vi "Lab Panel V5.29.vi"() -> ()   [LabVIEW 2013] (continued)
                  }
                }
              }
              event "RUN LAB01-2": Value Change {
                n578 = event-data() -> ("NewVal"=w843:bool)  [unwired: 1 in, 5 out]
                n579 = local write "run lab01-2"(w843) -> ()
                n580 = case shown="True" w843 {
                  tunnel: w849 -> [_ w887]
                  tunnel: w848 -> [_ w886]
                  tunnel: w846 -> [w851 w885]
                  tunnel: w847 -> [_ w884]
                  tunnel: w845 -> [_ w883]
                  tunnel: [w850 w882] -> w844
                  tunnel: w842 -> [_ w881]
                  tunnel: w841 -> [_ w880]
                  tunnel: w840 -> [_ w879]
                  tunnel: w839 -> [_ w877]
                  frame False {
                    # "stop test"
                    n581 = stacked-sequence {
                      tunnel: w851 -> [w860 _]
                      tunnel: [w852 _] -> w850
                      frame #0 {
                        n582 = local read "DISP LAB01-2"() -> (w859:T4)
                        n583 = Unbundle(w859) -> ("CYCLE"=w857:dbl, "MINS"=w858:dbl)  [unwired: 1 out]
                        n584 = case shown="\"CHART TEST\", Default" w860 {
                          tunnel: w858 -> [_ _ w867]
                          tunnel: w857 -> [w865 w866 _]
                          tunnel: [w865 w866 w867] -> w856
                          frame "CHART TEST", Default {
                          }
                          frame "CYCLE TEST" {
                          }
                          frame "T-RISE TEST" {
                          }
                        }
                        n585 = local read "TDMS LAB01-2"() -> (w864:refnum<k34>)
                        n586 = Build Array("STOPPED") -> (w861:string[])
                        n587 = Build Array(w856) -> (w855:dbl[])
                        n588 = TDMS Write(0:w864, 5:"TEST RESULT", 7:w861, 9:w855) -> (4:w853:refnum<k34>, 15:w854:errorcluster)  [unwired: 2 in, 2 out]
                        n589 = TDMS Close(8:w854, 11:w853) -> (0:w852:errorcluster)  [unwired: 1 out]
                      }
                      frame #1 {
                        n590 = local read "DISP LAB01-2"() -> (w871:T4)
                        n591 = stacked-sequence {
                          tunnel: "LAB01-2" -> [w873 w875]
                          frame #0 {
                            n592 = call "sub vi - defrag tdms v1.vi"("panel id"=w873) -> ("error out"=w872:errorcluster)  [unwired: 10 in]
                            n593 = local write "data file error"(w872) -> ()
                          }
                          frame #1 {
                            n594 = call "Save data file (stop) v3.vi"("panel id"=w875) -> ("network file save error"=w874:errorcluster)  [unwired: 9 in, 1 out]
                            n595 = local write "RESULT LAB01-2"(FALSE) -> ()
                            n596 = local write "data file error"(w874) -> ()
                          }
                        }
                        n597 = Bundle(cluster=w871, "STATUS"="STOP") -> (w869:T4)  [unwired: 2 in]
                        n598 = local write "DISP LAB01-2"(w869) -> ()
                      }
                    }
                  }
                  frame True {
                    n599 = local read "SIG LAB01-2"() -> (w878:T2)
                    n600 = stacked-sequence {
                      seq-local: [w889 _] -> [_ w893]
                      tunnel: w887 -> [_ w903]
                      tunnel: w886 -> [_ w902]
                      tunnel: w885 -> [_ w901]
                      tunnel: w884 -> [_ w900]
                      tunnel: w883 -> [_ w899]
                      tunnel: [_ w898] -> w882
                      tunnel: w881 -> [_ w897]
                      tunnel: w880 -> [_ w896]
                      tunnel: w879 -> [_ w895]
                      tunnel: w878 -> [w888 w894]
                      tunnel: w877 -> [_ w892]
                      frame #0 {
                        n601 = Unbundle(w888) -> ("AMPS"=w891:dbl)  [unwired: 4 out]
                        n602 = call "Check For Amps on v1.vi"("ID"="LAB01-2", "amps"=w891) -> ("amps"=w889:bool)  [unwired: 9 in]
                      }
                      frame #1 {
                        n603 = case shown="True" w893 {
                          tunnel: w903 -> [_ w916]
                          tunnel: w902 -> [_ w915]
                          tunnel: w901 -> [_ w914]
                          tunnel: w900 -> [_ w913]
                          tunnel: w899 -> [_ w912]
                          tunnel: [errorcluster {"status"=FALSE, "code"=0, "source"=""} ("error out") w911] -> w898
                          tunnel: w897 -> [_ w910]
                          tunnel: w896 -> [_ w909]
                          tunnel: w895 -> [_ w908]
                          tunnel: w894 -> [_ w907]
                          tunnel: w892 -> [_ w906]
                          frame False {
                            w904 = FALSE
                            n604 = local write "RUN LAB01-2"(w904) -> ()
                            n605 = local write "run lab01-2"(w904) -> ()
                          }
                          frame True {
                            n606 = stacked-sequence {
                              seq-local: [w917 _ _ _ _] -> [_ w941 _ _ _]
                              tunnel: w916 -> [w922 _ _ _ _]
                              tunnel: w915 -> [w919 _ _ _ _]
                              tunnel: w914 -> [w932 _ _ _ _]
                              tunnel: w913 -> [w925 _ _ _ _]
                              tunnel: w912 -> [w920 _ _ _ _]
                              tunnel: [_ w936 _ _ _] -> w911
                              tunnel: w910 -> [_ _ _ w963 _]
                              tunnel: w909 -> [_ _ _ w962 _]
                              tunnel: w908 -> [_ _ _ w961 _]
                              tunnel: w907 -> [_ _ _ _ _]
                              tunnel: w906 -> [_ _ _ _ w976]
                              frame #0 {
                                w918 = "\\"
                                n607 = local read "SET LAB01-2"() -> (w927:T5)
                                n608 = case shown="\"CYCLE TEST\"" w932 {
                                tunnel: ["L01-2-CHART TEST-" "L01-2-CYCLE TEST-" "L01-2-T-RISE TEST-"] -> w928
                                frame "CHART TEST", Default {
                                }
                                frame "CYCLE TEST" {
                                }
                                frame "T-RISE TEST" {
                                }
                                }
                                n609 = Unbundle(w927) -> ("DESCRIPTION"=w926:string)  [unwired: 4 out]
                                n610 = Concatenate Strings(w922, "\\", w920, w918, w919, w918) -> (w929:string)
                                n611 = String To Path(string=w929) -> (path=w931:path)
                                n612 = Concatenate Strings(w929, w928, w926, "-", w925, ".tdms") -> (w917:string)
                                n613 = Create Folder(path (use dialog)=w931) -> (error out=w930:errorcluster)  [unwired: 2 in, 2 out]
                                n614 = call <vilib>:"Clear Errors.vi"("error in (no error)"=w930) -> ()  [unwired: 6 in, 1 out]
                                n615 = global write "Global 1.vi" "LAB01-2 FILE"(w917) -> ()
                              }
                              frame #1 {
                                (unwired) FALSE
                                n616 = String To Path(string=w941) -> (path=w937:path)
                                n617 = TDMS Open(6:FALSE, 10:T21."create or replace" ("operation (0:open)"), 11:w937) -> (0:w936:errorcluster, 3:→"TDMS LAB01-2":refnum<k34>)  [unwired: 4 in]
                              }
                              frame #2 {
                                n618 = local read "SET LAB01-2"() -> (w947:T5)
                                n619 = local read "TDMS LAB01-2"() -> (w958:refnum<k34>)
                                n620 = Build Array("Testers Name", "Description", "Set Test Cycles", "T-Rise minutes", "T-Rise Deg C") -> (w948:string[])
                                n621 = Unbundle(w947) -> ("NAME"=w946:string, "DESCRIPTION"=w945:string, "CYCLES"=w944:dbl, "T-RISE mins"=w943:dbl, "T-RISE deg C"=w942:dbl)
                                n622 = Number To Decimal String(number=w944) -> (decimal integer string=w957:string)  [unwired: 1 in]
                                n623 = Number To Decimal String(number=w943) -> (decimal integer string=w956:string)  [unwired: 1 in]
                                n624 = Number To Decimal String(number=w942) -> (decimal integer string=w955:string)  [unwired: 1 in]
                                n625 = Build Array(w946, w945, w957, w956, w955) -> (w954:string[])
                                n626 = TDMS Set Properties(5:w954, 7:w948, 11:w958) -> ()  [unwired: 3 in, 4 out]
                              }
                              frame #3 {
                                n627 = local read "DISP LAB01-2"() -> (w960:T4)
                                n628 = Concatenate Strings("LAB01-2  ", w963) -> (w964:string)
                                n629 = Two Button Dialog(message=w964, 1:w961, 2:w962) -> (T button?=w966:bool)
                                n630 = case shown="True" w966 {
                                tunnel: w960 -> [w973 w974]
                                tunnel: [w973 w974] -> w970
                                tunnel: [w972 w975] -> w969
                                tunnel: [w971 w975] -> w968
                                frame False {
                                n631 = Unbundle(w973) -> ("CYCLE"=w972:dbl, "MINS"=w971:dbl)  [unwired: 1 out]
                                }
                                frame True {
                                w975 = 0.0
                                }
                                }
                                n632 = Bundle(cluster=w970, "CYCLE"=w969, "MINS"=w968, "STATUS"="RUN") -> (w959:T4)
                                n633 = local write "DISP LAB01-2"(w959) -> ()
                              }
                              frame #4 {
                                n634 = local read "TEMP START LAB01-2"() -> (w978:cluster{"TL":dbl, "TN":dbl})
                                n635 = Bundle(cluster=w978, "TL"=w976, "TN"=w976) -> (w977:cluster{"TL":dbl, "TN":dbl})
                                n636 = local write "TEMP START LAB01-2"(w977) -> ()
                              }
                            }
                          }
                        }
                      }
                    }
                  }
                }
              }
              event "RUN LAB02-1": Value Change {
                n637 = event-data() -> ("NewVal"=w984:bool)  [unwired: 1 in, 5 out]
                n638 = local read "SIG LAB02-1"() -> (w980:T2)
                n639 = case shown="True" w984 {
                  tunnel: w990 -> [_ w1028]
                  tunnel: w989 -> [_ w1027]
                  tunnel: w987 -> [w992 w1026]
                  tunnel: w988 -> [_ w1025]
                  tunnel: w986 -> [_ w1024]
                  tunnel: [w991 w1023] -> w985
                  tunnel: w983 -> [_ w1022]
                  tunnel: w982 -> [_ w1021]
                  tunnel: w981 -> [_ w1020]
                  tunnel: w980 -> [_ w1019]
                  tunnel: w979 -> [_ w1018]
                  frame False {
                    # "stop test"
                    n640 = stacked-sequence {
                      tunnel: w992 -> [w1001 _]
                      tunnel: [w993 _] -> w991
                      frame #0 {
                        n641 = local read "DISP LAB02-1"() -> (w1000:T4)
                        n642 = Unbundle(w1000) -> ("CYCLE"=w998:dbl, "MINS"=w999:dbl)  [unwired: 1 out]
                        n643 = case shown="\"CYCLE TEST\"" w1001 {
                          tunnel: w999 -> [_ _ w1008]
                          tunnel: w998 -> [w1006 w1007 _]
                          tunnel: [w1006 w1007 w1008] -> w997
                          frame "CHART TEST", Default {
                          }
                          frame "CYCLE TEST" {
                          }
                          frame "T-RISE TEST" {
                          }
                        }
                        n644 = local read "TDMS LAB02-1"() -> (w1005:refnum<k34>)
                        n645 = Build Array("STOPPED") -> (w1002:string[])
                        n646 = Build Array(w997) -> (w996:dbl[])
                        n647 = TDMS Write(0:w1005, 5:"TEST RESULT", 7:w1002, 9:w996) -> (4:w994:refnum<k34>, 15:w995:errorcluster)  [unwired: 2 in, 2 out]
                        n648 = TDMS Close(8:w995, 11:w994) -> (0:w993:errorcluster)  [unwired: 1 out]
                      }
                      frame #1 {
                        n649 = local read "DISP LAB02-1"() -> (w1012:T4)
                        n650 = stacked-sequence {
                          tunnel: "LAB02-1" -> [w1014 w1016]
                          frame #0 {
                            n651 = call "sub vi - defrag tdms v1.vi"("panel id"=w1014) -> ("error out"=w1013:errorcluster)  [unwired: 10 in]
                            n652 = local write "data file error"(w1013) -> ()
                          }
                          frame #1 {
                            n653 = local write "RESULT LAB02-1"(FALSE) -> ()
                            n654 = call "Save data file (stop) v3.vi"("panel id"=w1016) -> ("network file save error"=w1015:errorcluster)  [unwired: 9 in, 1 out]
                            n655 = local write "data file error"(w1015) -> ()
                          }
                        }
                        n656 = Bundle(cluster=w1012, "STATUS"="STOP") -> (w1010:T4)  [unwired: 2 in]
                        n657 = local write "DISP LAB02-1"(w1010) -> ()
                      }
                    }
                  }
                  frame True {
                    n658 = stacked-sequence {
                      seq-local: [w1030 _] -> [_ w1034]
                      tunnel: w1028 -> [_ w1044]
                      tunnel: w1027 -> [_ w1043]
                      tunnel: w1026 -> [_ w1042]
                      tunnel: w1025 -> [_ w1041]
                      tunnel: w1024 -> [_ w1040]
                      tunnel: [_ w1039] -> w1023
                      tunnel: w1022 -> [_ w1038]
                      tunnel: w1021 -> [_ w1037]
                      tunnel: w1020 -> [_ w1036]
                      tunnel: w1019 -> [w1029 w1035]
                      tunnel: w1018 -> [_ w1033]
                      frame #0 {
                        n659 = Unbundle(w1029) -> ("AMPS"=w1032:dbl)  [unwired: 4 out]
                        n660 = call "Check For Amps on v1.vi"("ID"="LAB02-1", "amps"=w1032) -> ("amps"=w1030:bool)  [unwired: 9 in]
                      }
                      frame #1 {
                        n661 = case shown="True" w1034 {
                          tunnel: w1044 -> [_ w1057]
                          tunnel: w1043 -> [_ w1056]
                          tunnel: w1042 -> [_ w1055]
                          tunnel: w1041 -> [_ w1054]
                          tunnel: w1040 -> [_ w1053]
                          tunnel: [errorcluster {"status"=FALSE, "code"=0, "source"=""} ("error out") w1052] -> w1039
                          tunnel: w1038 -> [_ w1051]
                          tunnel: w1037 -> [_ w1050]
                          tunnel: w1036 -> [_ w1049]
                          tunnel: w1035 -> [_ w1048]
                          tunnel: w1033 -> [_ w1047]
                          frame False {
                            w1046 = FALSE
                            n662 = local write "RUN LAB02-1"(w1046) -> ()
                            n663 = local write "run lab02-1"(w1046) -> ()
                          }
                          frame True {
                            n664 = stacked-sequence {
                              seq-local: [w1058 _ _ _ _] -> [_ w1082 _ _ _]
                              tunnel: w1057 -> [w1063 _ _ _ _]
                              tunnel: w1056 -> [w1060 _ _ _ _]
                              tunnel: w1055 -> [w1073 _ _ _ _]
                              tunnel: w1054 -> [w1066 _ _ _ _]
                              tunnel: w1053 -> [w1061 _ _ _ _]
                              tunnel: [_ w1077 _ _ _] -> w1052
                              tunnel: w1051 -> [_ _ _ w1103 _]
                              tunnel: w1050 -> [_ _ _ w1102 _]
                              tunnel: w1049 -> [_ _ _ w1101 _]
                              tunnel: w1048 -> [_ _ _ _ _]
                              tunnel: w1047 -> [_ _ _ _ w1117]
                              frame #0 {
                                w1059 = "\\"
                                n665 = local read "SET LAB02-1"() -> (w1068:T5)
                                n666 = case shown="\"CYCLE TEST\"" w1073 {
                                tunnel: ["L02-1-CHART TEST-" "L02-1-CYCLE TEST-" "L02-1-T-RISE TEST-"] -> w1069
                                frame "CHART TEST", Default {
                                }
                                frame "CYCLE TEST" {
                                }
                                frame "T-RISE TEST" {
                                }
                                }
                                n667 = Unbundle(w1068) -> ("DESCRIPTION"=w1067:string)  [unwired: 4 out]
                                n668 = Concatenate Strings(w1063, "\\", w1061, w1059, w1060, w1059) -> (w1070:string)
                                n669 = String To Path(string=w1070) -> (path=w1072:path)
                                n670 = Concatenate Strings(w1070, w1069, w1067, "-", w1066, ".tdms") -> (w1058:string)
                                n671 = Create Folder(path (use dialog)=w1072) -> (error out=w1071:errorcluster)  [unwired: 2 in, 2 out]
                                n672 = global write "Global 1.vi" "LAB02-1 FILE"(w1058) -> ()
                                n673 = call <vilib>:"Clear Errors.vi"("error in (no error)"=w1071) -> ()  [unwired: 6 in, 1 out]
                              }
                              frame #1 {
                                (unwired) FALSE
                                n674 = String To Path(string=w1082) -> (path=w1078:path)
                                n675 = TDMS Open(6:FALSE, 10:T21."create or replace" ("operation (0:open)"), 11:w1078) -> (0:w1077:errorcluster, 3:→"TDMS LAB02-1":refnum<k34>)  [unwired: 4 in]
                              }
                              frame #2 {
                                n676 = local read "SET LAB02-1"() -> (w1088:T5)
                                n677 = local read "TDMS LAB02-1"() -> (w1099:refnum<k34>)
                                n678 = Build Array("Testers Name", "Description", "Set Test Cycles", "T-Rise minutes", "T-Rise Deg C") -> (w1089:string[])
                                n679 = Unbundle(w1088) -> ("NAME"=w1087:string, "DESCRIPTION"=w1086:string, "CYCLES"=w1085:dbl, "T-RISE mins"=w1084:dbl, "T-RISE deg C"=w1083:dbl)
                                n680 = Number To Decimal String(number=w1085) -> (decimal integer string=w1098:string)  [unwired: 1 in]
                                n681 = Number To Decimal String(number=w1084) -> (decimal integer string=w1097:string)  [unwired: 1 in]
                                n682 = Number To Decimal String(number=w1083) -> (decimal integer string=w1096:string)  [unwired: 1 in]
                                n683 = Build Array(w1087, w1086, w1098, w1097, w1096) -> (w1095:string[])
                                n684 = TDMS Set Properties(5:w1095, 7:w1089, 11:w1099) -> ()  [unwired: 3 in, 4 out]
                              }
                              frame #3 {
                                n685 = local read "DISP LAB02-1"() -> (w1104:T4)
                                n686 = Concatenate Strings("LAB02-1  ", w1103) -> (w1105:string)
                                n687 = Two Button Dialog(message=w1105, 1:w1101, 2:w1102) -> (T button?=w1107:bool)
                                n688 = case shown="True" w1107 {
                                tunnel: w1104 -> [w1114 w1115]
                                tunnel: [w1114 w1115] -> w1111
                                tunnel: [w1113 w1116] -> w1110
                                tunnel: [w1112 w1116] -> w1109
                                frame False {
                                n689 = Unbundle(w1114) -> ("CYCLE"=w1113:dbl, "MINS"=w1112:dbl)  [unwired: 1 out]
                                }
                                frame True {
                                w1116 = 0.0
                                }
                                }
                                n690 = Bundle(cluster=w1111, "CYCLE"=w1110, "MINS"=w1109, "STATUS"="RUN") -> (w1100:T4)
                                n691 = local write "DISP LAB02-1"(w1100) -> ()
                              }
                              frame #4 {
                                n692 = local read "TEMP START LAB02-1"() -> (w1119:cluster{"TL":dbl, "TN":dbl})
                                n693 = Bundle(cluster=w1119, "TL"=w1117, "TN"=w1117) -> (w1118:cluster{"TL":dbl, "TN":dbl})
                                n694 = local write "TEMP START LAB02-1"(w1118) -> ()
                              }
                            }
                          }
                        }
                      }
                    }
                  }
                }
                n695 = local write "run lab02-1"(w984) -> ()
              }
              event "RUN LAB02-2": Value Change {
                n696 = event-data() -> ("NewVal"=w1124:bool)  [unwired: 1 in, 5 out]
                n697 = local write "run lab02-2"(w1124) -> ()
                n698 = case shown="True" w1124 {
                  tunnel: w1130 -> [_ w1168]
                  tunnel: w1129 -> [_ w1167]
                  tunnel: w1127 -> [w1132 w1166]
                  tunnel: w1128 -> [_ w1165]
                  tunnel: w1126 -> [_ w1164]
                  tunnel: [w1131 w1163] -> w1125
                  tunnel: w1123 -> [_ w1162]
                  tunnel: w1122 -> [_ w1161]
                  tunnel: w1121 -> [_ w1160]
                  tunnel: w1120 -> [_ w1158]
                  frame False {
                    # "stop test"
                    n699 = stacked-sequence {
                      tunnel: w1132 -> [w1141 _]
                      tunnel: [w1133 _] -> w1131
                      frame #0 {
                        n700 = local read "DISP LAB02-2"() -> (w1140:T4)
                        n701 = Unbundle(w1140) -> ("CYCLE"=w1138:dbl, "MINS"=w1139:dbl)  [unwired: 1 out]
                        n702 = case shown="\"CYCLE TEST\"" w1141 {
                          tunnel: w1139 -> [_ _ w1148]
                          tunnel: w1138 -> [w1146 w1147 _]
                          tunnel: [w1146 w1147 w1148] -> w1137
                          frame "CHART TEST", Default {
                          }
                          frame "CYCLE TEST" {
                          }
                          frame "T-RISE TEST" {
                          }
                        }
                        n703 = local read "TDMS LAB02-2"() -> (w1145:refnum<k34>)
                        n704 = Build Array("STOPPED") -> (w1142:string[])
                        n705 = Build Array(w1137) -> (w1136:dbl[])
                        n706 = TDMS Write(0:w1145, 5:"TEST RESULT", 7:w1142, 9:w1136) -> (4:w1134:refnum<k34>, 15:w1135:errorcluster)  [unwired: 2 in, 2 out]
                        n707 = TDMS Close(8:w1135, 11:w1134) -> (0:w1133:errorcluster)  [unwired: 1 out]
                      }
                      frame #1 {
                        n708 = local read "DISP LAB02-2"() -> (w1152:T4)
                        n709 = stacked-sequence {
                          tunnel: "LAB02-2" -> [w1154 w1156]
                          frame #0 {
                            n710 = call "sub vi - defrag tdms v1.vi"("panel id"=w1154) -> ("error out"=w1153:errorcluster)  [unwired: 10 in]
                            n711 = local write "data file error"(w1153) -> ()
                          }
                          frame #1 {
                            n712 = call "Save data file (stop) v3.vi"("panel id"=w1156) -> ("network file save error"=w1155:errorcluster)  [unwired: 9 in, 1 out]
                            n713 = local write "RESULT LAB02-2"(FALSE) -> ()
                            n714 = local write "data file error"(w1155) -> ()
                          }
                        }
                        n715 = Bundle(cluster=w1152, "STATUS"="STOP") -> (w1150:T4)  [unwired: 2 in]
                        n716 = local write "DISP LAB02-2"(w1150) -> ()
                      }
                    }
                  }
                  frame True {
                    n717 = local read "SIG LAB02-2"() -> (w1159:T2)
                    n718 = stacked-sequence {
                      seq-local: [w1170 _] -> [_ w1174]
                      tunnel: w1168 -> [_ w1184]
                      tunnel: w1167 -> [_ w1183]
                      tunnel: w1166 -> [_ w1182]
                      tunnel: w1165 -> [_ w1181]
                      tunnel: w1164 -> [_ w1180]
                      tunnel: [_ w1179] -> w1163
                      tunnel: w1162 -> [_ w1178]
                      tunnel: w1161 -> [_ w1177]
                      tunnel: w1160 -> [_ w1176]
                      tunnel: w1159 -> [w1169 w1175]
                      tunnel: w1158 -> [_ w1173]
                      frame #0 {
                        n719 = Unbundle(w1169) -> ("AMPS"=w1172:dbl)  [unwired: 4 out]
                        n720 = call "Check For Amps on v1.vi"("ID"="LAB02-2", "amps"=w1172) -> ("amps"=w1170:bool)  [unwired: 9 in]
                      }
                      frame #1 {
                        n721 = case shown="True" w1174 {
                          tunnel: w1184 -> [_ w1197]
                          tunnel: w1183 -> [_ w1196]
                          tunnel: w1182 -> [_ w1195]
                          tunnel: w1181 -> [_ w1194]
                          tunnel: w1180 -> [_ w1193]
                          tunnel: [errorcluster {"status"=FALSE, "code"=0, "source"=""} ("error out") w1192] -> w1179
                          tunnel: w1178 -> [_ w1191]
                          tunnel: w1177 -> [_ w1190]
                          tunnel: w1176 -> [_ w1189]
                          tunnel: w1175 -> [_ w1188]
                          tunnel: w1173 -> [_ w1187]
                          frame False {
                            w1185 = FALSE
                            n722 = local write "RUN LAB02-2"(w1185) -> ()
                            n723 = local write "run lab02-2"(w1185) -> ()
                          }
                          frame True {
                            n724 = stacked-sequence {
                              seq-local: [w1198 _ _ _ _] -> [_ w1222 _ _ _]
                              tunnel: w1197 -> [w1203 _ _ _ _]
                              tunnel: w1196 -> [w1200 _ _ _ _]
                              tunnel: w1195 -> [w1213 _ _ _ _]
                              tunnel: w1194 -> [w1206 _ _ _ _]
                              tunnel: w1193 -> [w1201 _ _ _ _]
                              tunnel: [_ w1217 _ _ _] -> w1192
                              tunnel: w1191 -> [_ _ _ w1243 _]
                              tunnel: w1190 -> [_ _ _ w1242 _]
                              tunnel: w1189 -> [_ _ _ w1241 _]
                              tunnel: w1188 -> [_ _ _ _ _]
                              tunnel: w1187 -> [_ _ _ _ w1257]
                              frame #0 {
                                w1199 = "\\"
                                n725 = local read "SET LAB02-2"() -> (w1208:T5)
                                n726 = case shown="\"CYCLE TEST\"" w1213 {
                                tunnel: ["L02-2-CHART TEST-" "L02-2-CYCLE TEST-" "L02-2-T-RISE TEST-"] -> w1209
                                frame "CHART TEST", Default {
                                }
                                frame "CYCLE TEST" {
                                }
                                frame "T-RISE TEST" {
                                }
                                }
                                n727 = Unbundle(w1208) -> ("DESCRIPTION"=w1207:string)  [unwired: 4 out]
                                n728 = Concatenate Strings(w1203, "\\", w1201, w1199, w1200, w1199) -> (w1210:string)
                                n729 = String To Path(string=w1210) -> (path=w1212:path)
                                n730 = Concatenate Strings(w1210, w1209, w1207, "-", w1206, ".tdms") -> (w1198:string)
                                n731 = Create Folder(path (use dialog)=w1212) -> (error out=w1211:errorcluster)  [unwired: 2 in, 2 out]
                                n732 = global write "Global 1.vi" "LAB02-2 FILE"(w1198) -> ()
                                n733 = call <vilib>:"Clear Errors.vi"("error in (no error)"=w1211) -> ()  [unwired: 6 in, 1 out]
                              }
                              frame #1 {
                                (unwired) FALSE
                                n734 = String To Path(string=w1222) -> (path=w1218:path)
                                n735 = TDMS Open(6:FALSE, 10:T21."create or replace" ("operation (0:open)"), 11:w1218) -> (0:w1217:errorcluster, 3:→"TDMS LAB02-2":refnum<k34>)  [unwired: 4 in]
                              }
                              frame #2 {
                                n736 = local read "SET LAB02-2"() -> (w1228:T5)
                                n737 = local read "TDMS LAB02-2"() -> (w1239:refnum<k34>)
                                n738 = Build Array("Testers Name", "Description", "Set Test Cycles", "T-Rise minutes", "T-Rise Deg C") -> (w1229:string[])
                                n739 = Unbundle(w1228) -> ("NAME"=w1227:string, "DESCRIPTION"=w1226:string, "CYCLES"=w1225:dbl, "T-RISE mins"=w1224:dbl, "T-RISE deg C"=w1223:dbl)
                                n740 = Number To Decimal String(number=w1225) -> (decimal integer string=w1238:string)  [unwired: 1 in]
                                n741 = Number To Decimal String(number=w1224) -> (decimal integer string=w1237:string)  [unwired: 1 in]
                                n742 = Number To Decimal String(number=w1223) -> (decimal integer string=w1236:string)  [unwired: 1 in]
                                n743 = Build Array(w1227, w1226, w1238, w1237, w1236) -> (w1235:string[])
                                n744 = TDMS Set Properties(5:w1235, 7:w1229, 11:w1239) -> ()  [unwired: 3 in, 4 out]
                              }
                              frame #3 {
                                n745 = local read "DISP LAB02-2"() -> (w1244:T4)
                                n746 = Concatenate Strings("LAB02-2  ", w1243) -> (w1245:string)
                                n747 = Two Button Dialog(message=w1245, 1:w1241, 2:w1242) -> (T button?=w1247:bool)
                                n748 = case shown="True" w1247 {
                                tunnel: w1244 -> [w1254 w1255]
                                tunnel: [w1254 w1255] -> w1251
                                tunnel: [w1253 w1256] -> w1250
                                tunnel: [w1252 w1256] -> w1249
                                frame False {
                                n749 = Unbundle(w1254) -> ("CYCLE"=w1253:dbl, "MINS"=w1252:dbl)  [unwired: 1 out]
                                }
                                frame True {
                                w1256 = 0.0
                                }
                                }
                                n750 = Bundle(cluster=w1251, "CYCLE"=w1250, "MINS"=w1249, "STATUS"="RUN") -> (w1240:T4)
                                n751 = local write "DISP LAB02-2"(w1240) -> ()
                              }
                              frame #4 {
                                n752 = local read "TEMP START LAB02-2"() -> (w1259:cluster{"TL":dbl, "TN":dbl})
                                n753 = Bundle(cluster=w1259, "TL"=w1257, "TN"=w1257) -> (w1258:cluster{"TL":dbl, "TN":dbl})
                                n754 = local write "TEMP START LAB02-2"(w1258) -> ()
                              }
                            }
                          }
                        }
                      }
                    }
                  }
                }
              }
              event "RUN LAB03-1": Value Change {
                n755 = event-data() -> ("NewVal"=w1264:bool)  [unwired: 1 in, 5 out]
                n756 = local write "run lab03-1"(w1264) -> ()
                n757 = case shown="True" w1264 {
                  tunnel: w1270 -> [_ w1308]
                  tunnel: w1269 -> [_ w1307]
                  tunnel: w1267 -> [w1272 w1306]
                  tunnel: w1268 -> [_ w1305]
                  tunnel: w1266 -> [_ w1304]
                  tunnel: [w1271 w1303] -> w1265
                  tunnel: w1263 -> [_ w1302]
                  tunnel: w1262 -> [_ w1301]
                  tunnel: w1261 -> [_ w1300]
                  tunnel: w1260 -> [_ w1298]
                  frame False {
                    # "stop test"
                    n758 = stacked-sequence {
                      tunnel: w1272 -> [w1281 _]
                      tunnel: [w1273 _] -> w1271
                      frame #0 {
                        n759 = local read "DISP LAB03-1"() -> (w1280:T4)
                        n760 = Unbundle(w1280) -> ("CYCLE"=w1278:dbl, "MINS"=w1279:dbl)  [unwired: 1 out]
                        n761 = case shown="\"CYCLE TEST\"" w1281 {
                          tunnel: w1279 -> [_ _ w1288]
                          tunnel: w1278 -> [w1286 w1287 _]
                          tunnel: [w1286 w1287 w1288] -> w1277
                          frame "CHART TEST", Default {
                          }
                          frame "CYCLE TEST" {
                          }
                          frame "T-RISE TEST" {
                          }
                        }
                        n762 = local read "TDMS LAB03-1"() -> (w1285:refnum<k34>)
                        n763 = Build Array("STOPPED") -> (w1282:string[])
                        n764 = Build Array(w1277) -> (w1276:dbl[])
                        n765 = TDMS Write(0:w1285, 5:"TEST RESULT", 7:w1282, 9:w1276) -> (4:w1274:refnum<k34>, 15:w1275:errorcluster)  [unwired: 2 in, 2 out]
                        n766 = TDMS Close(8:w1275, 11:w1274) -> (0:w1273:errorcluster)  [unwired: 1 out]
                      }
                      frame #1 {
                        n767 = local read "DISP LAB03-1"() -> (w1292:T4)
                        n768 = stacked-sequence {
                          tunnel: "LAB03-1" -> [w1294 w1296]
                          frame #0 {
                            n769 = call "sub vi - defrag tdms v1.vi"("panel id"=w1294) -> ("error out"=w1293:errorcluster)  [unwired: 10 in]
                            n770 = local write "data file error"(w1293) -> ()
                          }
                          frame #1 {
                            n771 = call "Save data file (stop) v3.vi"("panel id"=w1296) -> ("network file save error"=w1295:errorcluster)  [unwired: 9 in, 1 out]
                            n772 = local write "RESULT LAB03-1"(FALSE) -> ()
                            n773 = local write "data file error"(w1295) -> ()
                          }
                        }
                        n774 = Bundle(cluster=w1292, "STATUS"="STOP") -> (w1290:T4)  [unwired: 2 in]
                        n775 = local write "DISP LAB03-1"(w1290) -> ()
                      }
                    }
                  }
                  frame True {
                    n776 = local read "SIG LAB03-1"() -> (w1299:T2)
                    n777 = stacked-sequence {
                      seq-local: [w1310 _] -> [_ w1314]
                      tunnel: w1308 -> [_ w1324]
                      tunnel: w1307 -> [_ w1323]
                      tunnel: w1306 -> [_ w1322]
                      tunnel: w1305 -> [_ w1321]
                      tunnel: w1304 -> [_ w1320]
                      tunnel: [_ w1319] -> w1303
                      tunnel: w1302 -> [_ w1318]
                      tunnel: w1301 -> [_ w1317]
                      tunnel: w1300 -> [_ w1316]
                      tunnel: w1299 -> [w1309 w1315]
                      tunnel: w1298 -> [_ w1313]
                      frame #0 {
                        n778 = Unbundle(w1309) -> ("AMPS"=w1312:dbl)  [unwired: 4 out]
                        n779 = call "Check For Amps on v1.vi"("ID"="LAB03-1", "amps"=w1312) -> ("amps"=w1310:bool)  [unwired: 9 in]
                      }
                      frame #1 {
                        n780 = case shown="True" w1314 {
                          tunnel: w1324 -> [_ w1337]
                          tunnel: w1323 -> [_ w1336]
                          tunnel: w1322 -> [_ w1335]
                          tunnel: w1321 -> [_ w1334]
                          tunnel: w1320 -> [_ w1333]
                          tunnel: [errorcluster {"status"=FALSE, "code"=0, "source"=""} ("error out") w1332] -> w1319
                          tunnel: w1318 -> [_ w1331]
                          tunnel: w1317 -> [_ w1330]
                          tunnel: w1316 -> [_ w1329]
                          tunnel: w1315 -> [_ w1328]
                          tunnel: w1313 -> [_ w1327]
                          frame False {
                            w1325 = FALSE
                            n781 = local write "RUN LAB03-1"(w1325) -> ()
                            n782 = local write "run lab03-1"(w1325) -> ()
                          }
                          frame True {
                            n783 = stacked-sequence {
                              seq-local: [w1338 _ _ _ _] -> [_ w1362 _ _ _]
                              tunnel: w1337 -> [w1343 _ _ _ _]
                              tunnel: w1336 -> [w1340 _ _ _ _]
                              tunnel: w1335 -> [w1353 _ _ _ _]
                              tunnel: w1334 -> [w1346 _ _ _ _]
                              tunnel: w1333 -> [w1341 _ _ _ _]
                              tunnel: [_ w1357 _ _ _] -> w1332
                              tunnel: w1331 -> [_ _ _ w1382 _]
                              tunnel: w1330 -> [_ _ _ w1381 _]
                              tunnel: w1329 -> [_ _ _ w1380 _]
                              tunnel: w1328 -> [_ _ _ _ _]
                              tunnel: w1327 -> [_ _ _ _ w1397]
                              frame #0 {
                                w1339 = "\\"
                                n784 = local read "SET LAB03-1"() -> (w1348:T5)
                                n785 = case shown="\"T-RISE TEST\"" w1353 {
                                tunnel: ["L03-1-CHART TEST-" "L03-1-CYCLE TEST-" "L03-1-T-RISE TEST-"] -> w1349
                                frame "CHART TEST", Default {
                                }
                                frame "CYCLE TEST" {
                                }
                                frame "T-RISE TEST" {
                                }
                                }
                                n786 = Unbundle(w1348) -> ("DESCRIPTION"=w1347:string)  [unwired: 4 out]
                                n787 = Concatenate Strings(w1343, "\\", w1341, w1339, w1340, w1339) -> (w1350:string)
                                n788 = String To Path(string=w1350) -> (path=w1352:path)
                                n789 = Concatenate Strings(w1350, w1349, w1347, "-", w1346, ".tdms") -> (w1338:string)
                                n790 = Create Folder(path (use dialog)=w1352) -> (error out=w1351:errorcluster)  [unwired: 2 in, 2 out]
                                n791 = global write "Global 1.vi" "LAB03-1 FILE"(w1338) -> ()
                                n792 = call <vilib>:"Clear Errors.vi"("error in (no error)"=w1351) -> ()  [unwired: 6 in, 1 out]
                              }
                              frame #1 {
                                (unwired) FALSE
                                n793 = String To Path(string=w1362) -> (path=w1358:path)
                                n794 = TDMS Open(6:FALSE, 10:T21."create or replace" ("operation (0:open)"), 11:w1358) -> (0:w1357:errorcluster, 3:→"TDMS LAB03-1":refnum<k34>)  [unwired: 4 in]
                              }
                              frame #2 {
                                n795 = local read "SET LAB03-1"() -> (w1368:T5)
                                n796 = local read "TDMS LAB03-1"() -> (w1379:refnum<k34>)
                                n797 = Build Array("Testers Name", "Description", "Set Test Cycles", "T-Rise minutes", "T-Rise Deg C") -> (w1369:string[])
                                n798 = Unbundle(w1368) -> ("NAME"=w1367:string, "DESCRIPTION"=w1366:string, "CYCLES"=w1365:dbl, "T-RISE mins"=w1364:dbl, "T-RISE deg C"=w1363:dbl)
                                n799 = Number To Decimal String(number=w1365) -> (decimal integer string=w1378:string)  [unwired: 1 in]
                                n800 = Number To Decimal String(number=w1364) -> (decimal integer string=w1377:string)  [unwired: 1 in]
                                n801 = Number To Decimal String(number=w1363) -> (decimal integer string=w1376:string)  [unwired: 1 in]
                                n802 = Build Array(w1367, w1366, w1378, w1377, w1376) -> (w1375:string[])
                                n803 = TDMS Set Properties(5:w1375, 7:w1369, 11:w1379) -> ()  [unwired: 3 in, 4 out]
                              }
                              frame #3 {
                                n804 = local read "DISP LAB03-1"() -> (w1384:T4)
                                n805 = Concatenate Strings("LAB03-1  ", w1382) -> (w1385:string)
                                n806 = Two Button Dialog(message=w1385, 1:w1380, 2:w1381) -> (T button?=w1387:bool)
                                n807 = case shown="True" w1387 {
                                tunnel: w1384 -> [w1394 w1395]
                                tunnel: [w1394 w1395] -> w1391
                                tunnel: [w1393 w1396] -> w1390
                                tunnel: [w1392 w1396] -> w1389
                                frame False {
                                n808 = Unbundle(w1394) -> ("CYCLE"=w1393:dbl, "MINS"=w1392:dbl)  [unwired: 1 out]
                                }
                                frame True {
                                w1396 = 0.0
                                }
                                }
                                n809 = Bundle(cluster=w1391, "CYCLE"=w1390, "MINS"=w1389, "STATUS"="RUN") -> (w1383:T4)
                                n810 = local write "DISP LAB03-1"(w1383) -> ()
                              }
                              frame #4 {
                                n811 = local read "TEMP START LAB03-1"() -> (w1399:cluster{"TL":dbl, "TN":dbl})
                                n812 = Bundle(cluster=w1399, "TL"=w1397, "TN"=w1397) -> (w1398:cluster{"TL":dbl, "TN":dbl})
                                n813 = local write "TEMP START LAB03-1"(w1398) -> ()
                              }
                            }
                          }
                        }
                      }
                    }
                  }
                }
              }
              event "RUN LAB03-2": Value Change {
                n814 = event-data() -> ("NewVal"=w1404:bool)  [unwired: 1 in, 5 out]
                n815 = local write "run lab03-2"(w1404) -> ()
                n816 = case shown="True" w1404 {
                  tunnel: w1410 -> [_ w1448]
                  tunnel: w1409 -> [_ w1447]
                  tunnel: w1407 -> [w1412 w1446]
                  tunnel: w1408 -> [_ w1445]
                  tunnel: w1406 -> [_ w1444]
                  tunnel: [w1411 w1443] -> w1405
                  tunnel: w1403 -> [_ w1442]
                  tunnel: w1402 -> [_ w1441]
                  tunnel: w1401 -> [_ w1440]
                  tunnel: w1400 -> [_ w1438]
                  frame False {
                    # "stop test"
                    n817 = stacked-sequence {
                      tunnel: w1412 -> [w1421 _]
                      tunnel: [w1413 _] -> w1411
                      frame #0 {
                        n818 = local read "DISP LAB03-2"() -> (w1420:T4)
                        n819 = Unbundle(w1420) -> ("CYCLE"=w1418:dbl, "MINS"=w1419:dbl)  [unwired: 1 out]
                        n820 = case shown="\"CYCLE TEST\"" w1421 {
                          tunnel: w1419 -> [_ _ w1428]
                          tunnel: w1418 -> [w1426 w1427 _]
                          tunnel: [w1426 w1427 w1428] -> w1417
                          frame "CHART TEST", Default {
                          }
                          frame "CYCLE TEST" {
                          }
                          frame "T-RISE TEST" {
                          }
                        }
                        n821 = local read "TDMS LAB03-2"() -> (w1425:refnum<k34>)
                        n822 = Build Array("STOPPED") -> (w1422:string[])
                        n823 = Build Array(w1417) -> (w1416:dbl[])
                        n824 = TDMS Write(0:w1425, 5:"TEST RESULT", 7:w1422, 9:w1416) -> (4:w1414:refnum<k34>, 15:w1415:errorcluster)  [unwired: 2 in, 2 out]
                        n825 = TDMS Close(8:w1415, 11:w1414) -> (0:w1413:errorcluster)  [unwired: 1 out]
                      }
                      frame #1 {
                        n826 = local read "DISP LAB03-2"() -> (w1432:T4)
                        n827 = stacked-sequence {
                          tunnel: "LAB03-2" -> [w1434 w1436]
                          frame #0 {
                            n828 = call "sub vi - defrag tdms v1.vi"("panel id"=w1434) -> ("error out"=w1433:errorcluster)  [unwired: 10 in]
                            n829 = local write "data file error"(w1433) -> ()
                          }
                          frame #1 {
                            n830 = call "Save data file (stop) v3.vi"("panel id"=w1436) -> ("network file save error"=w1435:errorcluster)  [unwired: 9 in, 1 out]
                            n831 = local write "RESULT LAB03-2"(FALSE) -> ()
                            n832 = local write "data file error"(w1435) -> ()
                          }
                        }
                        n833 = Bundle(cluster=w1432, "STATUS"="STOP") -> (w1430:T4)  [unwired: 2 in]
                        n834 = local write "DISP LAB03-2"(w1430) -> ()
                      }
                    }
                  }
                  frame True {
                    n835 = local read "SIG LAB03-2"() -> (w1439:T2)
                    n836 = stacked-sequence {
                      seq-local: [w1450 _] -> [_ w1454]
                      tunnel: w1448 -> [_ w1464]
                      tunnel: w1447 -> [_ w1463]
                      tunnel: w1446 -> [_ w1462]
                      tunnel: w1445 -> [_ w1461]
                      tunnel: w1444 -> [_ w1460]
                      tunnel: [_ w1459] -> w1443
                      tunnel: w1442 -> [_ w1458]
                      tunnel: w1441 -> [_ w1457]
                      tunnel: w1440 -> [_ w1456]
                      tunnel: w1439 -> [w1449 w1455]
                      tunnel: w1438 -> [_ w1453]
                      frame #0 {
                        n837 = Unbundle(w1449) -> ("AMPS"=w1452:dbl)  [unwired: 4 out]
                        n838 = call "Check For Amps on v1.vi"("ID"="LAB03-2", "amps"=w1452) -> ("amps"=w1450:bool)  [unwired: 9 in]
                      }
                      frame #1 {
                        n839 = case shown="True" w1454 {
                          tunnel: w1464 -> [_ w1477]
                          tunnel: w1463 -> [_ w1476]
                          tunnel: w1462 -> [_ w1475]
                          tunnel: w1461 -> [_ w1474]
                          tunnel: w1460 -> [_ w1473]
                          tunnel: [errorcluster {"status"=FALSE, "code"=0, "source"=""} ("error out") w1472] -> w1459
                          tunnel: w1458 -> [_ w1471]
                          tunnel: w1457 -> [_ w1470]
                          tunnel: w1456 -> [_ w1469]
                          tunnel: w1455 -> [_ w1468]
                          tunnel: w1453 -> [_ w1467]
                          frame False {
                            w1465 = FALSE
                            n840 = local write "RUN LAB03-2"(w1465) -> ()
                            n841 = local write "run lab03-2"(w1465) -> ()
                          }
                          frame True {
                            n842 = stacked-sequence {
                              seq-local: [w1478 _ _ _ _] -> [_ w1502 _ _ _]
                              tunnel: w1477 -> [w1483 _ _ _ _]
                              tunnel: w1476 -> [w1480 _ _ _ _]
                              tunnel: w1475 -> [w1493 _ _ _ _]
                              tunnel: w1474 -> [w1486 _ _ _ _]
                              tunnel: w1473 -> [w1481 _ _ _ _]
                              tunnel: [_ w1497 _ _ _] -> w1472
                              tunnel: w1471 -> [_ _ _ w1523 _]
                              tunnel: w1470 -> [_ _ _ w1522 _]
                              tunnel: w1469 -> [_ _ _ w1521 _]
                              tunnel: w1468 -> [_ _ _ _ _]
                              tunnel: w1467 -> [_ _ _ _ w1537]
                              frame #0 {
                                w1479 = "\\"
                                n843 = local read "SET LAB03-2"() -> (w1488:T5)
                                n844 = case shown="\"T-RISE TEST\"" w1493 {
                                tunnel: ["L03-2-CHART TEST-" "L03-2-CYCLE TEST-" "L03-2-T-RISE TEST-"] -> w1489
